vi "Drive Immediate.vi"(6 "Center Setpoint":dbl, 7 "Description":string, 8 "Command Info In":T1, 9 "Deadband Value":dbl=0.01, 10 "Right Setpoint":dbl, 11 "Left Setpoint":dbl) -> (0 "Command Info Out":T1)   [LabVIEW 2018]
doc: "Often used for joystick control, this VI checks to see that the joystick axes are outside the deadband and updates the motors appropriately."
uses:
  <vilib>/Rock Robotics/WPI/Framework/Command Status Info.ctl
  <vilib>/Rock Robotics/WPI/Framework/Completion Status.ctl
  <vilib>/Rock Robotics/WPI/Framework/Completion Notifier.ctl
  Implementation/Drive Setpoints.ctl
  Implementation/Drive Operations.ctl
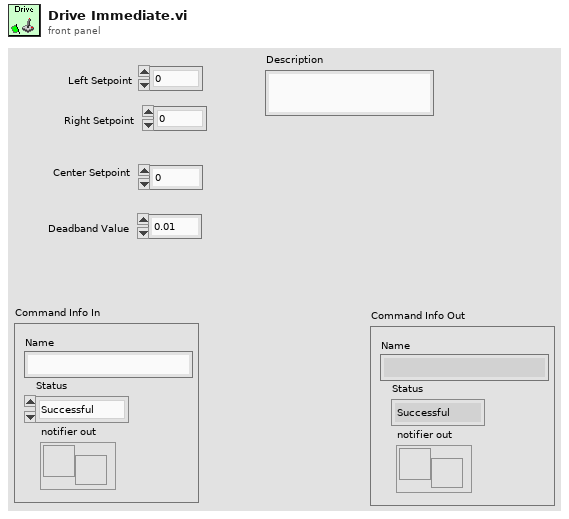
[diagram p1: front panel]
types:
  T1 = typedef "Command Status Info.ctl" = cluster{"Name":string, "Status":T2, "notifier out":T3}
  T2 = typedef "Completion Status.ctl" = enum16{"Successful", "Aborted", "Incomplete"}
  T3 = typedef "Completion Notifier.ctl" = refnum<notifier>
  T4 = typedef "Drive Setpoints.ctl" = cluster{"Operation":T5, "Left Setpoint":dbl, "Right Setpoint":dbl, "Duration":dbl, "Center Setpoint":dbl}
  T5 = typedef "Drive Operations.ctl" = enum16{"Reserve", "Read Current", "Immediate", "Drive for Time", "Drive for Distance"}
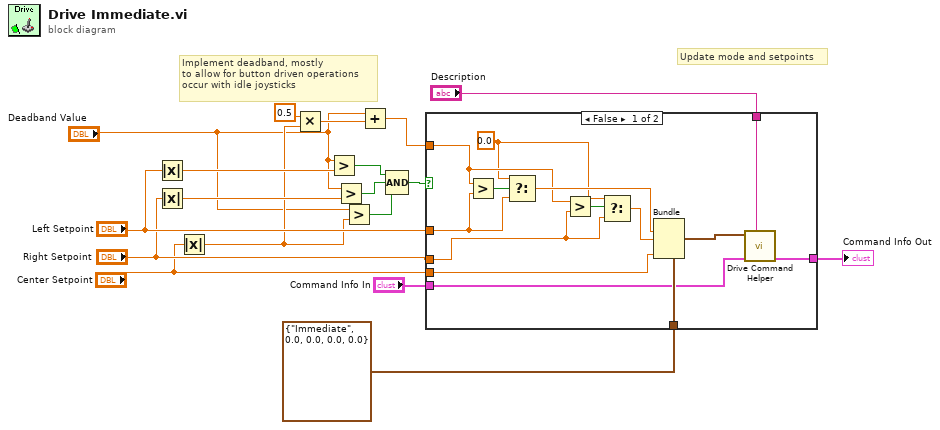
[diagram p0: block diagram]
diagram:
  # "Implement deadband, mostly\nto allow for button driven operations\noccur with idle joysticks"
  # "Update mode and setpoints"
  n1 = Absolute Value(x="Left Setpoint") -> (abs(x)=w18:dbl)
  n2 = Absolute Value(x="Right Setpoint") -> (abs(x)=w12:dbl)
  n3 = Absolute Value(x="Center Setpoint") -> (abs(x)=w4:dbl)
  n4 = Multiply(x=0.5, y=w4) -> (x*y=w5:dbl)
  n5 = Greater?(x="Deadband Value", y=w18) -> (0:w7:bool)
  n6 = Greater?(x="Deadband Value", y=w12) -> (0:w8:bool)
  n7 = Greater?(x="Deadband Value", y=w4) -> (0:w9:bool)
  n8 = Add(x="Deadband Value", y=w5) -> (x+y=w1:dbl)
  n9 = Compound Arithmetic op=AND(w7, w8, w9) -> (w6:bool)
  n10 = case shown="False" w6 {
    tunnel: "Left Setpoint" -> [w24 _]
    tunnel: T4 {"Operation"=enum."Immediate", "Left Setpoint"=0.0, "Right Setpoint"=0.0, "Duration"=0.0, "Center Setpoint"=0.0} ("SubSystem Data") -> [w32 _]
    tunnel: [w31 w33] -> w17
    tunnel: "Command Info In" -> [w30 w33]
    tunnel: "Description" -> [w28 _]
    tunnel: "Right Setpoint" -> [w23 _]
    tunnel: "Center Setpoint" -> [w27 _]
    tunnel: w1 -> [w20 _]
    frame False {
      w19 = 0.0 ("t")
      n11 = Greater?(x=w20, y=w24) -> (0:w26:bool)
      n12 = Select(t=w19, s=w26, f=w24) -> (s? t:f=w21:dbl)
      n13 = Greater?(x=w20, y=w23) -> (0:w25:bool)
      n14 = Select(t=w19, s=w25, f=w23) -> (s? t:f=w22:dbl)
      n15 = Bundle(cluster=w32, "Left Setpoint"=w21, "Right Setpoint"=w22, "Center Setpoint"=w27) -> (w29:T4)  [unwired: 2 in]
      n16 = call "Drive Command Helper.vi"("Description"=w28, "Command Info In"=w30, "SubSystem Data"=w29) -> ("Command Info Out"=w31:T1)  [unwired: 6 in, 2 out]
    }
    frame True {
    }
  }
  "Command Info Out" <- w17
